vi "Rolling Average.vi"(10 "New Value":dbl, 11 "Old Array":dbl[](array[numeric])) -> (2 "Calculated Value":dbl, 3 "New Array":dbl[](array[numeric]))   [LabVIEW 2018, in "Support Library.lvlib"]
uses:
  Support Library.lvlib
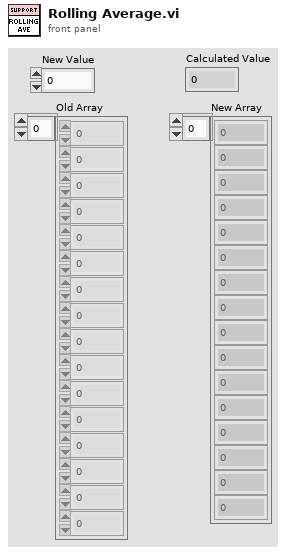
[diagram p1: front panel]
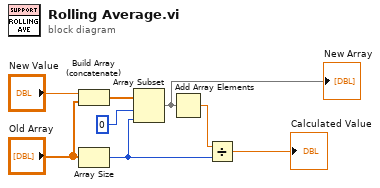
[diagram p0: block diagram]
diagram:
  n1 = Build Array (concatenate)("New Value", "Old Array") -> (w3:dbl[])
  n2 = Array Size(array="Old Array") -> (size(s)=w5:i32)
  n3 = Array Subset(array=w3, index=0, length=w5) -> (w1:dbl[])
  "New Array" <- w1
  n4 = Add Array Elements(numeric array=w1) -> (sum=w2:dbl)
  n5 = Divide(x=w2, y=w5) -> (x/y=→"Calculated Value":dbl)
